vi "MainControlGUI.vi"() -> ()   [LabVIEW 2017]
uses:
  <vilib>/Platform/TimedLoop/XDataNode/timing_clust.ctl
  <vilib>/Platform/TimedLoop/XDataNode/nitl_modes.ctl
  <vilib>/Platform/TimedLoop/XDataNode/wakeup.ctl
  <vilib>/platform/TimedLoop/XDataNode/XDataNode.xnode
  <vilib>/Platform/TimedLoop/XDataNode/XDNodeRunTimeDep.lvlib
panel:
  in  "LM335Z Raw (V)":dbl
  out "LM335Z Temp (C)":dbl format="%#_13g"
  in  "MCP9700 Raw (V)":dbl
  out "MCP9700 Temp (C)":dbl format="%#_13g"
  in  "Update Rate (ms)":dbl=1.0 min=10.0
  in  "STOP":bool
  in  "TMP36 Raw (V)":dbl
  out "TMP36 Temp (C)":dbl format="%#_13g"
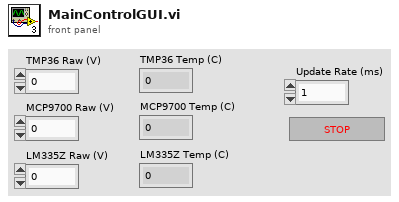
[diagram p1: front panel]
types:
  T1 = typedef "XDNodeRunTimeDep.lvlib/timing_clust.ctl" = cluster{"Expected End [f-1]":u64, "Actual End [f-1]":u64, "Finished Late? [f-1]":bool, "Expected End [i-1]":u64, "Actual End [i-1]":u64, "Finished Late? [i-1]":bool, "Expected Start [i]":u64, "Actual Start [i]":u64, "Expected Start [f]":u64, "Actual Start [f]":u64, "Source Name":string, "Structure Name":string, "Period":i64, "Deadline":i64, "Offset":i64, "Start":i64, "Priority":i32, "Timeout":i32, "Mode":T2, "Wakeup Reason":T3, "Error":errorcluster, "Source Type":string, "Secondary Source Type":string, "Global End Time":u64, "Global Start Time":u64, "Frame Duration":u64, "Iteration Duration":u64, "Assigned CPU":i32, "I/O Scan Engine Mode":u32}
  T2 = typedef "XDNodeRunTimeDep.lvlib/nitl_modes.ctl" = enum32{"No Change", "Process missed periods, maintain original phase", "Discard missed periods, maintain original phase", "Process missed periods, ignore original phase", "Discard missed periods, ignore original phase"}
  T3 = typedef "XDNodeRunTimeDep.lvlib/wakeup.ctl" = enum32{"Normal", "Aborted", "Asynchronous wakeup", "Timing source error", "Timed loop error", "Timeout"}
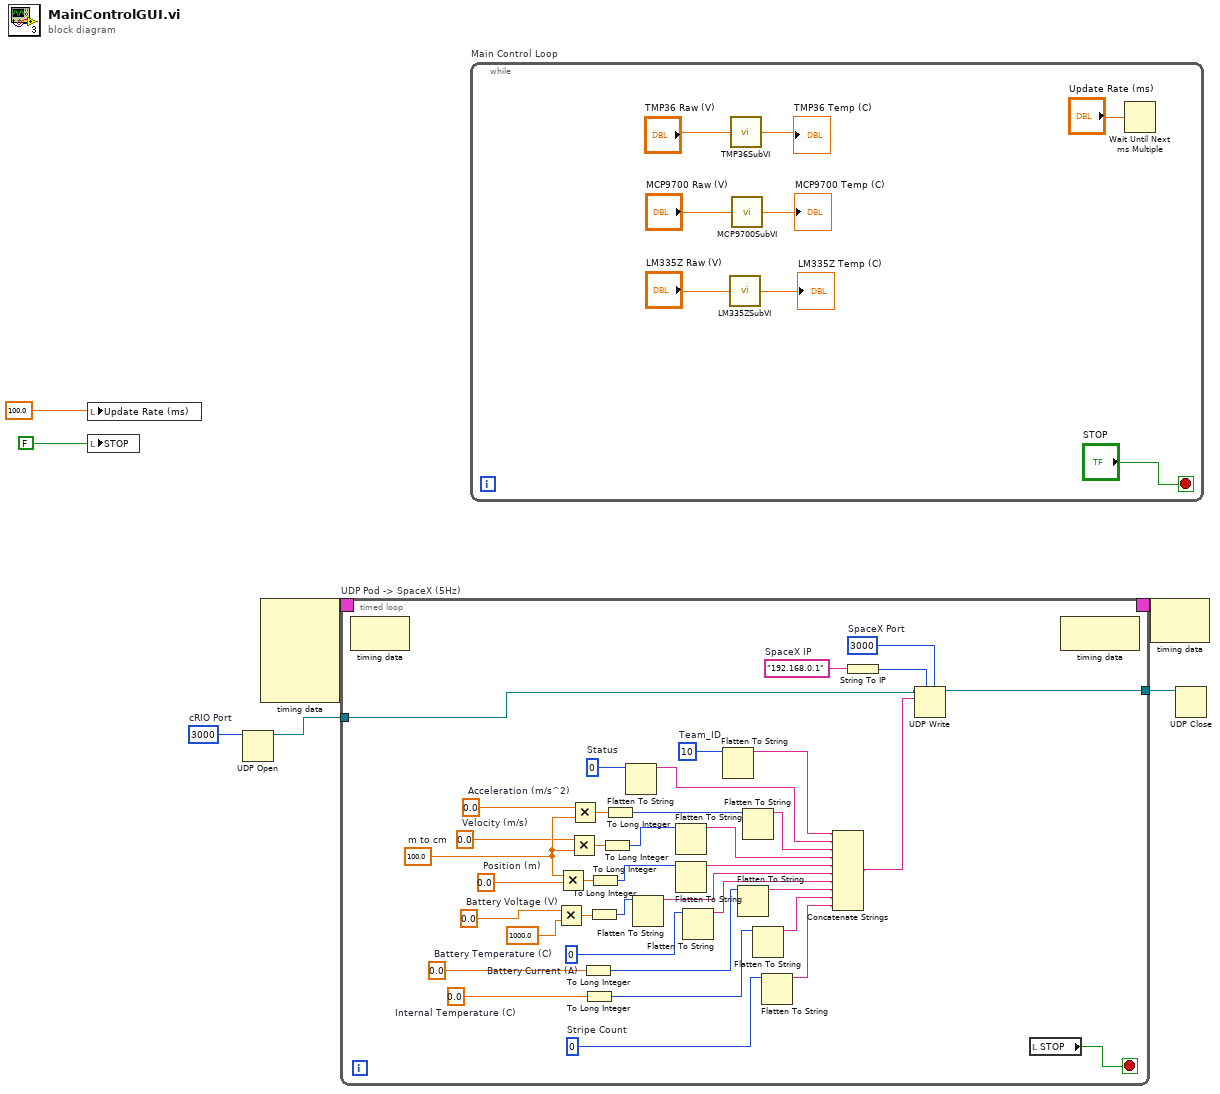
[diagram p0: block diagram]
diagram:
  w5 = u32 3000  # cRIO Port
  n1 = local write "Update Rate (ms)"(100.0) -> ()
  n2 = local write "STOP"(FALSE) -> ()
  n3 = UDP Open(11:w5) -> (port=w4:refnum<k16>)  [unwired: 4 in, 2 out]
  n4 = node-c288() -> (w7:T1)  [unwired: 5 in]
  n5 = timed-loop "UDP Pod -> SpaceX (5Hz)" {
    timing: w7 -> [_]
    timing-out: [_] -> w6
    tunnel: w4 -> [w17]
    tunnel: [w16] -> w3
    stop <- w15 stop-if-true
    w8 = 0.0  # Internal Temperature (C)
    w12 = 0.0  # Position (m)
    w11 = 0.0  # Velocity (m/s)
    w10 = 0.0  # Battery Voltage (V)
    w9 = 0.0  # Battery Temperature (C)
    w13 = 0.0  # Acceleration (m/s^2)
    w14 = 0  # Status
    w18 = u32 0  # Stripe Count
    w24 = 0  # Battery Current (A)
    w46 = 100.0  # m to cm
    w35 = u8 10  # Team_ID
    w37 = u16 3000  # SpaceX Port
    w40 = "192.168.0.1"  # SpaceX IP
    n6 = node-c288() -> ()  [unwired: 1 in, 1 out]
    n7 = Multiply(x=w10, y=1000.0) -> (x*y=w42:dbl)
    n8 = Multiply(x=w46, y=w12) -> (x*y=w43:dbl)
    n9 = Multiply(x=w11, y=w46) -> (x*y=w44:dbl)
    n10 = Multiply(x=w13, y=w46) -> (x*y=w45:dbl)
    n11 = To Long Integer(number=w9) -> (32bit integer=w22:i32)
    n12 = To Long Integer(number=w8) -> (32bit integer=w20:i32)
    n13 = To Long Integer(number=w42) -> (32bit integer=w26:i32)
    n14 = To Long Integer(number=w43) -> (32bit integer=w28:i32)
    n15 = To Long Integer(number=w44) -> (32bit integer=w30:i32)
    n16 = To Long Integer(number=w45) -> (32bit integer=w33:i32)
    n17 = Flatten To String(anything=w14) -> (data string=w34:string)  [unwired: 3 in, 2 out]
    n18 = Flatten To String(anything=w26) -> (data string=w27:string)  [unwired: 3 in, 2 out]
    n19 = Flatten To String(anything=w30) -> (data string=w31:string)  [unwired: 3 in, 2 out]
    n20 = Flatten To String(anything=w28) -> (data string=w29:string)  [unwired: 3 in, 2 out]
    n21 = Flatten To String(anything=w24) -> (data string=w25:string)  [unwired: 3 in, 2 out]
    n22 = Flatten To String(anything=w35) -> (data string=w36:string)  [unwired: 3 in, 2 out]
    n23 = Flatten To String(anything=w22) -> (data string=w23:string)  [unwired: 3 in, 2 out]
    n24 = Flatten To String(anything=w33) -> (data string=w32:string)  [unwired: 3 in, 2 out]
    n25 = Flatten To String(anything=w20) -> (data string=w21:string)  [unwired: 3 in, 2 out]
    n26 = Flatten To String(anything=w18) -> (data string=w19:string)  [unwired: 3 in, 2 out]
    n27 = Concatenate Strings(w36, w34, w32, w31, w29, w27, w25, w23, w21, w19) -> (w39:string)
    n28 = String To IP(1:w40) -> (0:w38:u32)
    n29 = UDP Write(address=w38, port or service name=w37, connection ID=w17, data in=w39) -> (3:w16:refnum<k16>)  [unwired: 2 in, 1 out]
    n30 = local read "STOP"() -> (w15:bool)
    n31 = node-c288() -> ()  [unwired: 1 in, 1 out]
  }
  n32 = while "Main Control Loop" {
    stop <- "STOP" stop-if-true
    n33 = call "LM335ZSubVI.vi"("Raw Input (V)"="LM335Z Raw (V)") -> ("Temperature (C)"=→"LM335Z Temp (C)":dbl)
    n34 = call "TMP36SubVI.vi"("Raw Input (V)"="TMP36 Raw (V)") -> ("Temperature (C)"=→"TMP36 Temp (C)":dbl)
    n35 = call "MCP9700SubVI.vi"("Raw Input (V)"="MCP9700 Raw (V)") -> ("Temperature (C)"=→"MCP9700 Temp (C)":dbl)
    n36 = Wait Until Next ms Multiple(millisecond multiple="Update Rate (ms)") -> ()  [unwired: 1 out]
  }
  n37 = node-c288(w6) -> ()  [unwired: 1 out]
  n38 = UDP Close(connection ID=w3) -> ()  [unwired: 1 in, 2 out]
